vi "Menu-Start Acq EOC.vi"(11 "Menu in":refnum<k9>) -> ()   [LabVIEW 2016, in "CML UI.lvlib"]
uses:
  CML UI.lvlib
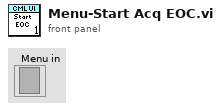
[diagram p1: front panel]
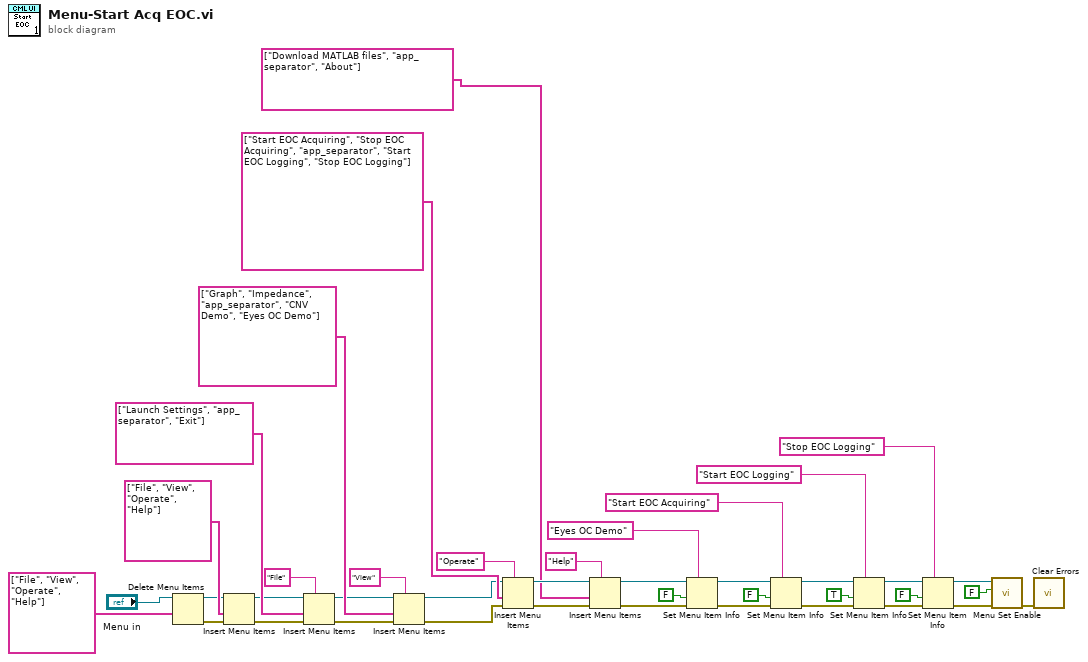
[diagram p0: block diagram]
diagram:
  n1 = Delete Menu Items(7:string[] ["File", "View", "Operate", "Help"] ("L10n_item tags 1"), 9:"Menu in") -> (0:w17:errorcluster, 3:w18:refnum<k9>)  [unwired: 2 in]
  n2 = Insert Menu Items(6:w17, 7:string[] ["File", "View", "Operate", "Help"] ("L10n_item tags 1"), 9:w18) -> (0:w30:errorcluster, 3:w28:refnum<k9>)  [unwired: 3 in, 1 out]
  n3 = Insert Menu Items(5:"File" ("L10n_menu tag"), 6:w30, 7:string[] ["Launch Settings", "app_separator", "Exit"] ("L10n_item tags 2"), 9:w28) -> (0:w35:errorcluster, 3:w34:refnum<k9>)  [unwired: 2 in, 1 out]
  n4 = Insert Menu Items(5:"View" ("L10n_menu tag"), 6:w35, 7:string[] ["Graph", "Impedance", "app_separator", "CNV Demo", "Eyes OC Demo"] ("L10n_item tags 2"), 9:w34) -> (0:w39:errorcluster, 3:w38:refnum<k9>)  [unwired: 2 in, 1 out]
  n5 = Insert Menu Items(5:"Operate" ("L10n_menu tag"), 6:w39, 7:string[] ["Start EOC Acquiring", "Stop EOC Acquiring", "app_separator", "Start EOC Logging", "Stop EOC Logging"] ("L10n_item tags 2"), 9:w38) -> (0:w25:errorcluster, 3:w26:refnum<k9>)  [unwired: 2 in, 1 out]
  n6 = Insert Menu Items(5:"Help" ("L10n_menu tag"), 6:w25, 7:string[] ["Download MATLAB files", "app_separator", "About"] ("L10n_item tags 2"), 9:w26) -> (0:w22:errorcluster, 3:w24:refnum<k9>)  [unwired: 2 in, 1 out]
  n7 = Set Menu Item Info(7:"Eyes OC Demo" ("item tag"), 8:w22, 9:FALSE ("enabled"), 11:w24) -> (0:w11:errorcluster, 3:w12:refnum<k9>)  [unwired: 3 in]
  n8 = Set Menu Item Info(7:"Start EOC Acquiring" ("item tag"), 8:w11, 9:FALSE ("enabled"), 11:w12) -> (0:w9:errorcluster, 3:w10:refnum<k9>)  [unwired: 3 in]
  n9 = Set Menu Item Info(7:"Start EOC Logging" ("item tag"), 8:w9, 9:TRUE ("enabled"), 11:w10) -> (0:w7:errorcluster, 3:w8:refnum<k9>)  [unwired: 3 in]
  n10 = Set Menu Item Info(7:"Stop EOC Logging" ("item tag"), 8:w7, 9:FALSE ("enabled"), 11:w8) -> (0:w5:errorcluster, 3:w4:refnum<k9>)  [unwired: 3 in]
  n11 = call "Menu Set Enable.vi"("error in (no error)"=w5, "enabled ?"=FALSE, "Menu in"=w4) -> ("error out"=w3:errorcluster)  [unwired: 7 in, 1 out]
  n12 = call <vilib>:"Clear Errors.vi"("error in (no error)"=w3) -> ()  [unwired: 5 in, 2 out]
